vi "超简计算器.vi"() -> ()   [LabVIEW 2018]
panel:
  in  "除":bool
  in  "乘":bool
  in  "减":bool
  in  "加":bool
  out "结果":dbl
  in  "输入2":dbl
  in  "输入1":dbl
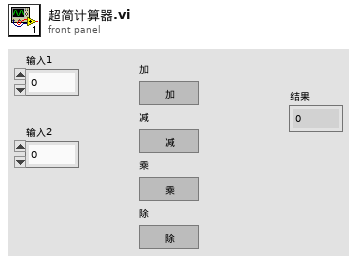
[diagram p1: front panel]
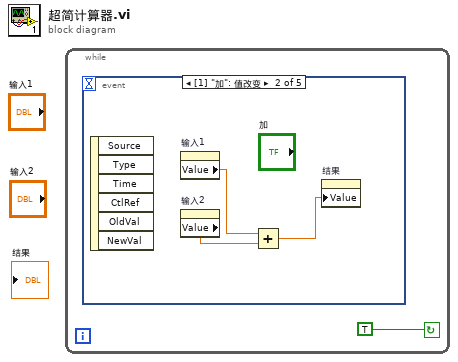
[diagram p0: block diagram]
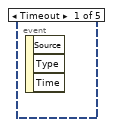
[diagram p2: hidden frame]
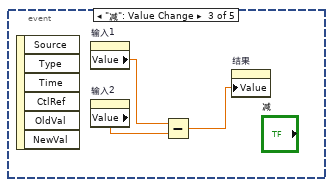
[diagram p3: hidden frame]
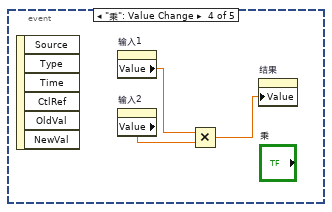
[diagram p4: hidden frame]
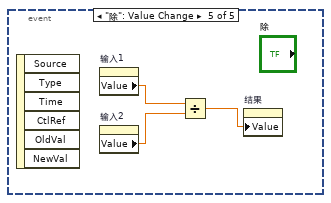
[diagram p5: hidden frame]
diagram:
  n1 = while {
    stop <- TRUE ("停止") continue-if-true
    n2 = event shown="[1] \"加\": 值改变" {
      selector: _ -> [_ _ _ _ _]
      dyn-events: _ -> [_ _ _ _ _]
      timeout: _ -> [_ _ _ _ _]
      event Timeout {
        n3 = event-data() -> ()  [unwired: 1 in, 3 out]
      }
      event "加": Value Change {
        n4 = event-data() -> ()  [unwired: 1 in, 6 out]
        n5 = property on="输入1" class="DigNum (严格)"() -> ("Value"=w4:dbl)  [unwired: 2 in, 2 out]
        n6 = property on="输入2" class="DigNum (严格)"() -> ("Value"=w2:dbl)  [unwired: 2 in, 2 out]
        n7 = Add(x=w4, y=w2) -> (x+y=w3:dbl)
        n8 = property on="结果" class="DigNum (严格)"("Value"=w3) -> ()  [unwired: 2 in, 2 out]
      }
      event "减": Value Change {
        n9 = event-data() -> ()  [unwired: 1 in, 6 out]
        n10 = property on="输入1" class="DigNum (严格)"() -> ("Value"=w7:dbl)  [unwired: 2 in, 2 out]
        n11 = property on="输入2" class="DigNum (严格)"() -> ("Value"=w5:dbl)  [unwired: 2 in, 2 out]
        n12 = Subtract(x=w7, y=w5) -> (x-y=w6:dbl)
        n13 = property on="结果" class="DigNum (严格)"("Value"=w6) -> ()  [unwired: 2 in, 2 out]
      }
      event "乘": Value Change {
        n14 = event-data() -> ()  [unwired: 1 in, 6 out]
        n15 = property on="输入1" class="DigNum (严格)"() -> ("Value"=w10:dbl)  [unwired: 2 in, 2 out]
        n16 = property on="输入2" class="DigNum (严格)"() -> ("Value"=w9:dbl)  [unwired: 2 in, 2 out]
        n17 = Multiply(x=w10, y=w9) -> (x*y=w8:dbl)
        n18 = property on="结果" class="DigNum (严格)"("Value"=w8) -> ()  [unwired: 2 in, 2 out]
      }
      event "除": Value Change {
        n19 = event-data() -> ()  [unwired: 1 in, 6 out]
        n20 = property on="输入1" class="DigNum (严格)"() -> ("Value"=w13:dbl)  [unwired: 2 in, 2 out]
        n21 = property on="输入2" class="DigNum (严格)"() -> ("Value"=w12:dbl)  [unwired: 2 in, 2 out]
        n22 = Divide(x=w13, y=w12) -> (x/y=w11:dbl)
        n23 = property on="结果" class="DigNum (严格)"("Value"=w11) -> ()  [unwired: 2 in, 2 out]
      }
    }
  }
